vi "电信1801-2018012704-杜兴安-虚拟仪器作业4.vi"() -> ()   [LabVIEW 2020]
uses:
  <vilib>/Waveform/DWDTOps.llb/DWDT Binary U16 to Digital.vi
  <vilib>/Utility/file.llb/Read Delimited Spreadsheet (DBL).vi
  <vilib>/Utility/file.llb/Write Delimited Spreadsheet (DBL).vi
  <vilib>/Analysis/NI_AALBase.lvlib
panel:
  out "波形图":dbl[](graph)
  out "sin":dynamicdata(graph)
  out "波形图 2":dbl[](graph)
  out "温度 3":dbl
  out "日期 2":string
  out "时间 2":string
  in  "温度 2":dbl
  out "温度":dbl
  out "温度计":dbl(slide) scale=0.0..100.0
  out "日期":string
  out "时间":string
  out "数组":dbl[][](array[numeric])
  out "数字波形图 2":digitalwaveform(graph)
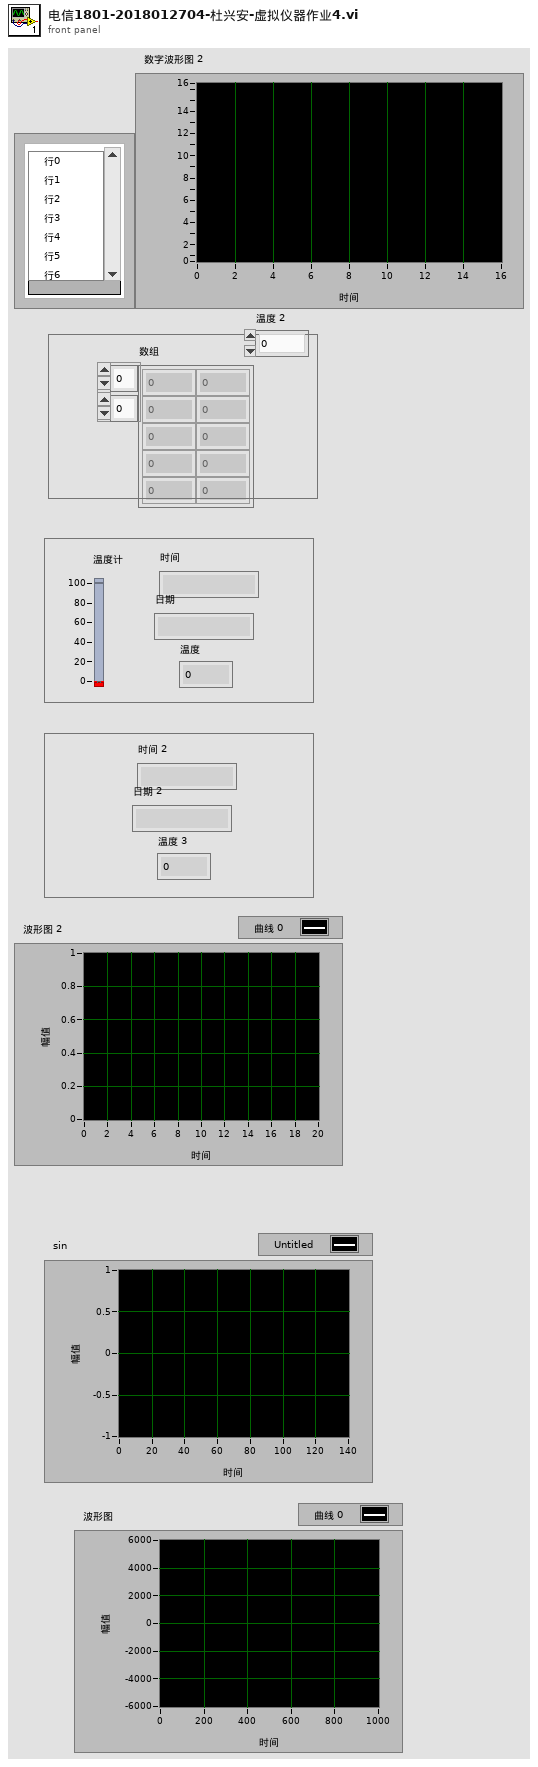
[diagram p1: front panel]
types:
  T1 = enum16{"open", "replace", "create", "open or create", "replace or create", "replace or create with confirmation"}
  T2 = cluster{dbl, "date string":string, "time string":string}
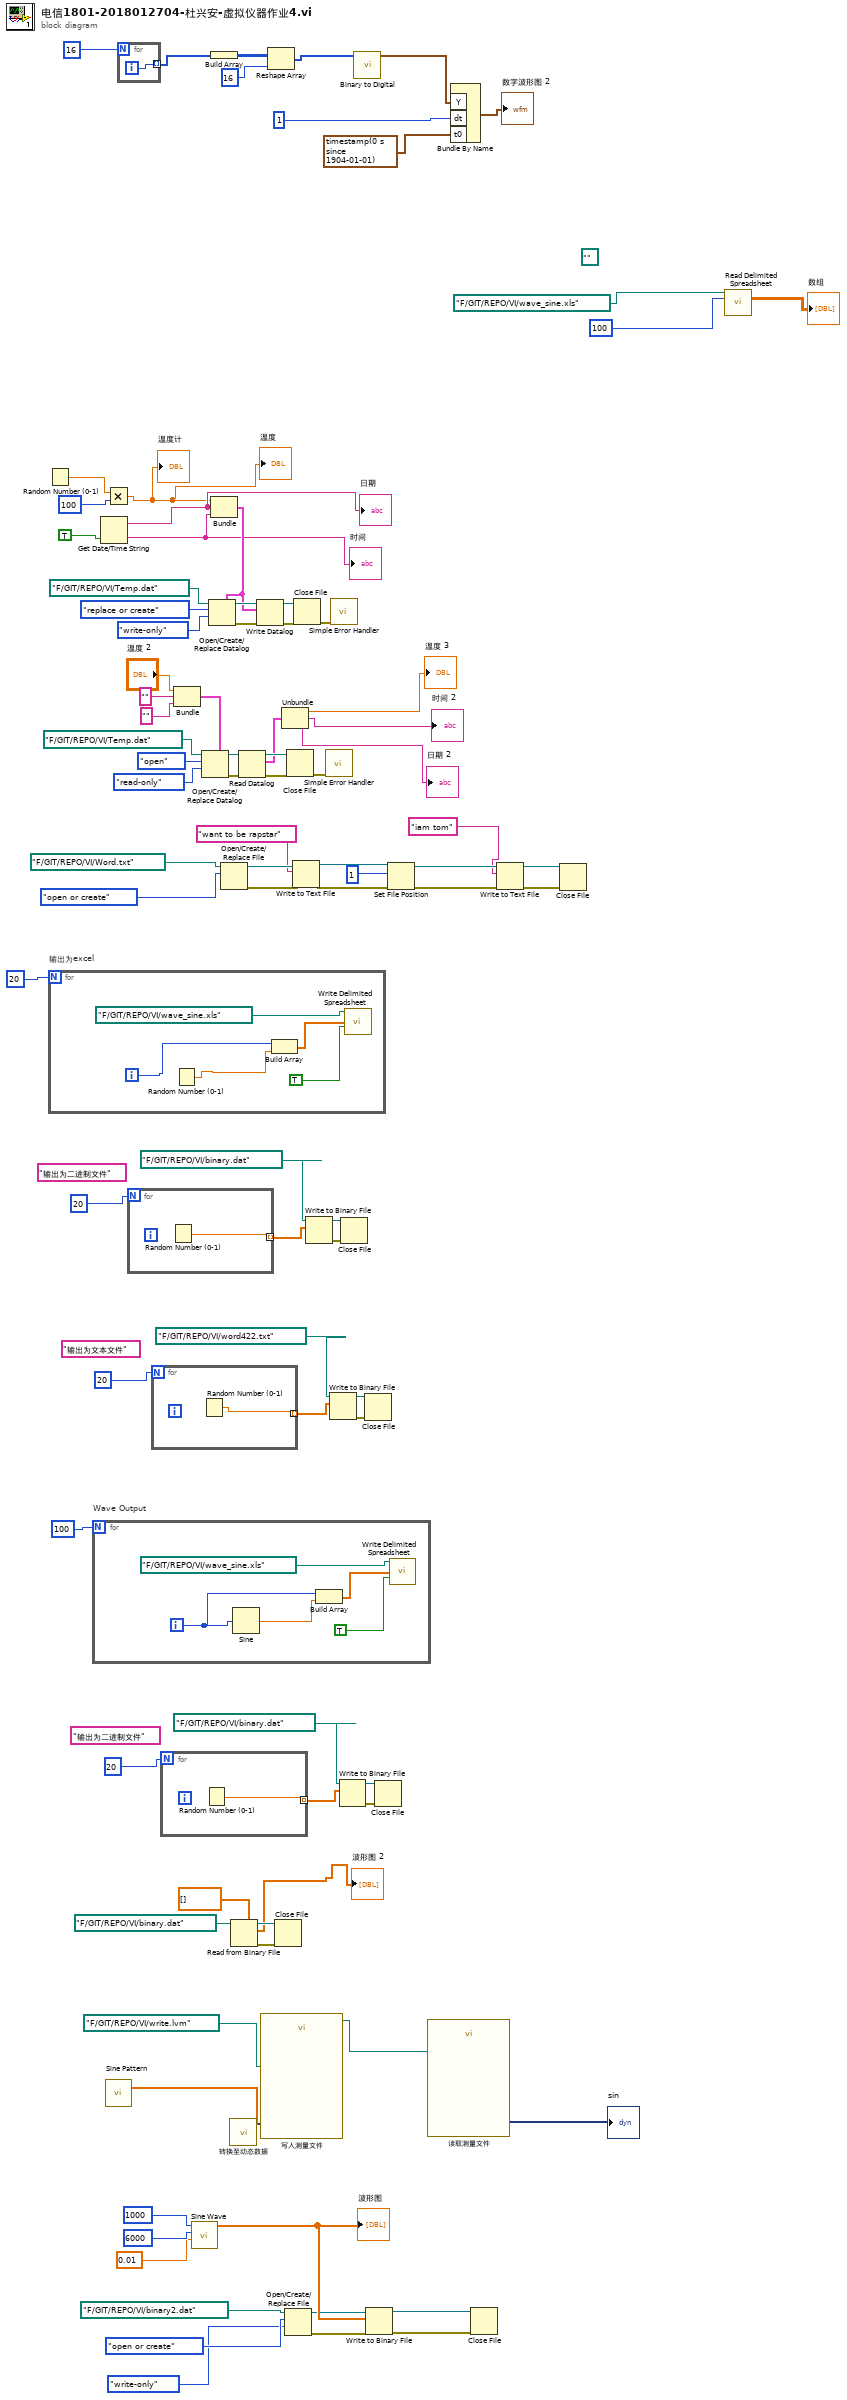
[diagram p0: block diagram]
diagram:
  (unwired) "输出为二进制文件"
  (unwired) "输出为文本文件"
  (unwired) "输出为二进制文件"
  (unwired) path ""
  n1 = Random Number (0-1)() -> (number: 0 to 1=w58:dbl)
  n2 = for "输出为excel" {
    N: 20 -> [_]
    i -> [w99]
    n3 = Random Number (0-1)() -> (number: 0 to 1=w95:dbl)
    n4 = Build Array(w99, w95) -> (w96:dbl[])
    n5 = call-poly <vilib>:"Write Delimited Spreadsheet.vi"("file path (dialog if empty)"=path "F:/GIT/REPO/VI/wave_sine.xls", "1D data"=w96, "append to file? (new file:F)"=TRUE) -> ()  [unwired: 11 in, 2 out]
  }
  n6 = for "Wave Output" {
    N: 100 -> [_]
    i -> [w104]
    n7 = Sine(x=w104) -> (sin(x)=w103:dbl)
    n8 = Build Array(w104, w103) -> (w100:dbl[])
    n9 = call-poly <vilib>:"Write Delimited Spreadsheet.vi"("file path (dialog if empty)"=path "F:/GIT/REPO/VI/wave_sine.xls", "1D data"=w100, "append to file? (new file:F)"=TRUE) -> ()  [unwired: 11 in, 2 out]
  }
  n10 = Get Date/Time String(want seconds? (F)=TRUE) -> (date string=w71:string, time string=w72:string)  [unwired: 2 in]
  "时间" <- w72
  "日期" <- w71
  n11 = Multiply(x=w58, y=100) -> (x*y=w57:dbl)
  "温度计" <- w57
  "温度" <- w57
  n12 = call <vilib>:"Sine Pattern.vi"() -> ("Sinusoidal Pattern"=w15:dbl[])  [unwired: 4 in, 1 out]
  n13 = for {
    N: 16 -> [_]
    tunnel: [w105] -> w92 mode=indexing
    i -> [w105]
  }
  n14 = for {
    N: 20 -> [_]
    tunnel: [w106] -> w34 mode=indexing
    n15 = Random Number (0-1)() -> (number: 0 to 1=w106:dbl)
  }
  n16 = for {
    N: 20 -> [_]
    tunnel: [w107] -> w29 mode=indexing
    n17 = Random Number (0-1)() -> (number: 0 to 1=w107:dbl)
  }
  n18 = for {
    N: 20 -> [_]
    tunnel: [w108] -> w23 mode=indexing
    n19 = Random Number (0-1)() -> (number: 0 to 1=w108:dbl)
  }
  n20 = Bundle("温度 2"="温度 2", "", "") -> (w62:cluster{"温度 2":dbl, string, string})  [unwired: 1 in]
  n21 = call <vilib>:"Sine Wave.vi"("samples"=1000, "amplitude"=6000, "frequency"=0.01) -> ("sine wave"=w8:dbl[])  [unwired: 2 in, 2 out]
  "波形图" <- w8
  n22 = Open/Create/Replace Datalog(5:w62, 9:enum16{"read/write", "read-only", "write-only"}."read-only" ("权限(0:read/write)"), 10:T1."open" ("操作(0:open)"), 11:path "F:/GIT/REPO/VI/Temp.dat" ("数据记录路径（使用对话框）")) -> (0:w66:errorcluster, 3:w61:refnum<k1>)  [unwired: 2 in, 1 out]
  n23 = Build Array(w92) -> (w91:i32[][])
  n24 = Bundle(w57, "date string"=w71, "time string"=w72) -> (w73:T2)  [unwired: 1 in]
  n25 = Open/Create/Replace Datalog(5:w73, 9:enum16{"read/write", "read-only", "write-only"}."write-only" ("权限(0:read/write)"), 10:T1."replace or create" ("操作(0:open)"), 11:path "F:/GIT/REPO/VI/Temp.dat" ("数据记录路径（使用对话框）")) -> (0:w77:errorcluster, 3:w78:refnum<k1>)  [unwired: 2 in, 1 out]
  n26 = Open/Create/Replace File(file path (use dialog)=path "F:/GIT/REPO/VI/Word.txt" ("数据记录路径（使用对话框）"), operation (0:open)=T1."open or create" ("操作(0:open)")) -> (refnum out=w49:refnum<file>, error out=w47:errorcluster)  [unwired: 4 in, 1 out]
  n27 = call "转换至动态数据"("Array"=w15) -> ("Dynamic Data Type"=w14:dynamicdata)  [unwired: 3 in]
  n28 = Read from Binary File(5:dbl[] [], 11:path "F:/GIT/REPO/VI/binary.dat" ("文件（使用对话框）")) -> (0:w18:errorcluster, 2:→"波形图 2":dbl[], 3:w19:refnum<file>)  [unwired: 4 in, 1 out]
  n29 = Read Datalog(4:w66, 7:w61) -> (0:w64:errorcluster, 2:w60:cluster{"温度 2":dbl, string, string}, 3:w65:refnum<k1>)  [unwired: 1 in]
  n30 = Write Datalog(4:w77, 6:w73, 7:w78) -> (0:w75:errorcluster, 3:w76:refnum<k1>)
  n31 = call "写入测量文件"("Signals"=w14, "Filename"=path "F:/GIT/REPO/VI/write.lvm" ("文件（使用对话框）")) -> ("Filename Out"=w13:path)  [unwired: 15 in, 2 out]
  n32 = Reshape Array(w91, 16) -> (w89:i32[])
  n33 = Close File(refnum=w19, error in=w18) -> ()  [unwired: 2 out]
  n34 = Unbundle(w60) -> ("温度 2"=→"温度 3":dbl, →"时间 2":string, →"日期 2":string)
  n35 = Open/Create/Replace File(file path (use dialog)=path "F:/GIT/REPO/VI/binary2.dat", operation (0:open)=T1."open or create" ("操作(0:open)"), access (0:read/write)=enum16{"read/write", "read-only", "write-only"}."write-only" ("权限(0:read/write)")) -> (refnum out=w4:refnum<file>, error out=w3:errorcluster)  [unwired: 3 in, 1 out]
  n36 = Close File(refnum=w65, error in=w64) -> (error out=w70:errorcluster)  [unwired: 1 out]
  n37 = Write to Text File(file (use dialog)=w49, text="want to be rapstar", error in=w47) -> (refnum out=w46:refnum<file>, error out=w45:errorcluster)  [unwired: 1 in, 1 out]
  n38 = Close File(refnum=w76, error in=w75) -> (error out=w82:errorcluster)  [unwired: 1 out]
  n39 = Write to Binary File(file (use dialog)=path "F:/GIT/REPO/VI/binary.dat" ("文件（使用对话框）"), data=w34) -> (refnum out=w35:refnum<file>, error out=w36:errorcluster)  [unwired: 4 in, 1 out]
  n40 = call <vilib>:"Simple Error Handler.vi"("error in (no error)"=w70) -> ()  [unwired: 4 in, 5 out]
  n41 = Write to Binary File(file (use dialog)=path "F:/GIT/REPO/VI/word422.txt" ("文件（使用对话框）"), data=w29) -> (refnum out=w30:refnum<file>, error out=w31:errorcluster)  [unwired: 4 in, 1 out]
  n42 = call <vilib>:"Simple Error Handler.vi"("error in (no error)"=w82) -> ()  [unwired: 4 in, 5 out]
  n43 = Write to Binary File(file (use dialog)=path "F:/GIT/REPO/VI/binary.dat" ("文件（使用对话框）"), data=w23) -> (refnum out=w24:refnum<file>, error out=w25:errorcluster)  [unwired: 4 in, 1 out]
  n44 = Close File(refnum=w35, error in=w36) -> ()  [unwired: 2 out]
  n45 = call-poly <vilib>:"Binary to Digital.vi"("binary array"=w89) -> ("digital waveform"=w86:digitalwaveform)  [unwired: 9 in, 1 out]
  n46 = Close File(refnum=w30, error in=w31) -> ()  [unwired: 2 out]
  n47 = Write to Binary File(file (use dialog)=w4, data=w8, error in=w3) -> (refnum out=w1:refnum<file>, error out=w2:errorcluster)  [unwired: 3 in, 1 out]
  n48 = Close File(refnum=w24, error in=w25) -> ()  [unwired: 2 out]
  n49 = Set File Position(offset (in bytes) (0)=1, refnum=w46, error in=w45) -> (refnum out=w43:refnum<file>, error out=w42:errorcluster)  [unwired: 1 in]
  n50 = call "读取测量文件"("Filename"=w13) -> ("Signals"=→"sin":dynamicdata)  [unwired: 5 in, 5 out]
  n51 = Bundle By Name ("创建波形")("Y"=w86, "dt"=1, "t0"=timestamp(0 s since 1904-01-01)) -> (→"数字波形图 2":digitalwaveform)  [unwired: 1 in]
  n52 = Close File(refnum=w1, error in=w2) -> ()  [unwired: 2 out]
  n53 = Write to Text File(file (use dialog)=w43, text="iam tom", error in=w42) -> (refnum out=w40:refnum<file>, error out=w39:errorcluster)  [unwired: 1 in, 1 out]
  n54 = Close File(refnum=w40, error in=w39) -> ()  [unwired: 2 out]
  n55 = call-poly <vilib>:"Read Delimited Spreadsheet.vi"("file path (dialog if empty)"=path "F:/GIT/REPO/VI/wave_sine.xls", "number of rows (all:-1)"=100) -> ("all rows"=→"数组":dbl[][])  [unwired: 8 in, 5 out]
